vi "随机数出数.vi"(10 "百分比":dbl, 11 "输入":dbl) -> (3 "输出":dbl)   [LabVIEW 2016, in "仿真数据.lvlib"]
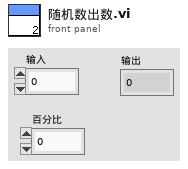
[diagram p1: front panel]
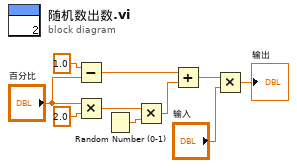
[diagram p0: block diagram]
diagram:
  n1 = Subtract(x=1.0, y="百分比") -> (x-y=w5:dbl)
  n2 = Multiply(x="百分比", y=2.0) -> (x*y=w2:dbl)
  n3 = Random Number (0-1)() -> (number: 0 to 1=w6:dbl)
  n4 = Multiply(x=w2, y=w6) -> (x*y=w7:dbl)
  n5 = Add(x=w5, y=w7) -> (x+y=w8:dbl)
  n6 = Multiply(x=w8, y="输入") -> (x*y=→"输出":dbl)
